vi "get-bit-array-from-payload.vi"(4 "CAN frame":T1 {"payload" format="%x"; "timestamp" format="%<%.7X\n%x>T"; "type" items=["CAN Data"=0, "CAN Remote"=1, "CAN Bus Error"=2, "J1939 Data"=192, "Delay"=224, "Log Trigger"=225, "Start Trigger"=226]; "identifier" format="%x"}) -> (1 "Array":bool[](array[boolean]))   [LabVIEW 2015]
uses:
  <vilib>/xnet/xnet.llb/XNET Frame CAN.ctl
  <vilib>/xnet/xnet.llb/XNET Frame Type CAN.ctl
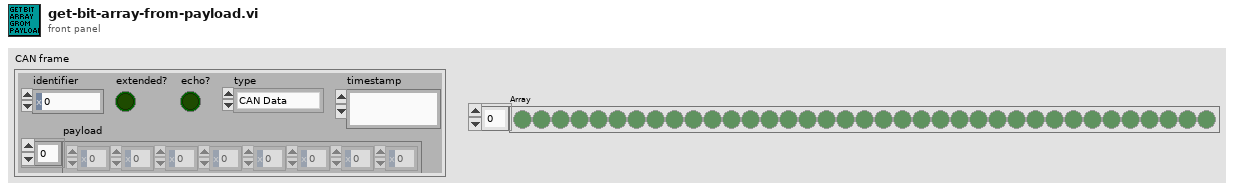
[diagram p1: front panel]
types:
  T1 = typedef "XNET Frame CAN.ctl" = cluster{"timestamp":timestamp, "payload":u8[], "identifier":u32, "type":T2, "extended?":bool, "echo?":bool}
  T2 = typedef "XNET Frame Type CAN.ctl" = u8
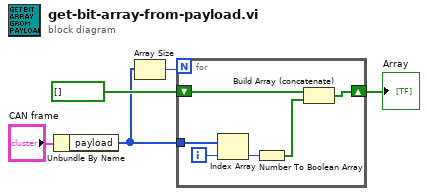
[diagram p0: block diagram]
diagram:
  n1 = Unbundle By Name("CAN frame") -> ("payload"=w1:u8[])
  n2 = Array Size(array=w1) -> (size(s)=w2:i32)
  n3 = for {
    N: w2 -> [_]
    tunnel: w1 -> [w11]
    shift-right: [w8] -> w4
    shift-left: bool[] [] -> [w9]
    i -> [w6]
    n4 = Index Array(array=w11, index=w6) -> (element=w10:u8)
    n5 = Number To Boolean Array(number=w10) -> (Boolean array=w7:bool[])
    n6 = Build Array (concatenate)(w9, w7) -> (w8:bool[])
  }
  "Array" <- w4
